vi "GE5565 Write (U64) Cluster.vi"(6 "timeout (1000 ms)":u32=1000, 8 "error in (no error)":errorcluster, 9 "buffer":dbl[](array[numeric]), 10 "offset (0)":u32, 11 "VMIC reference in":T1) -> (0 "error out":errorcluster, 3 "VMIC reference out":T1)   [LabVIEW 2015]
uses:
  <vilib>/Instr/_visa.llb/Select Event Type.ctl
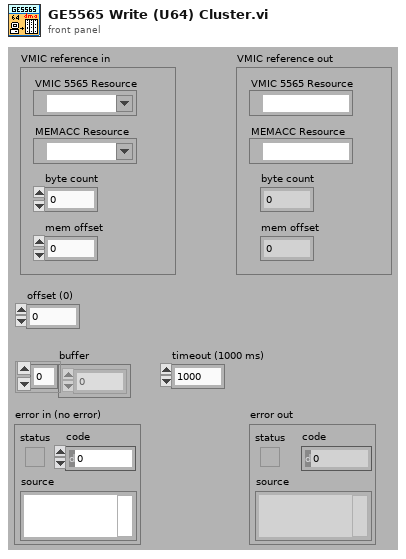
[diagram p1: front panel]
types:
  T1 = cluster{"VMIC 5565 Resource":refnum<visa-resource-name>, "MEMACC Resource":refnum<visa-resource-name>, "byte count":u32, "mem offset":u32}
  T2 = typedef "Select Event Type.ctl" = u32
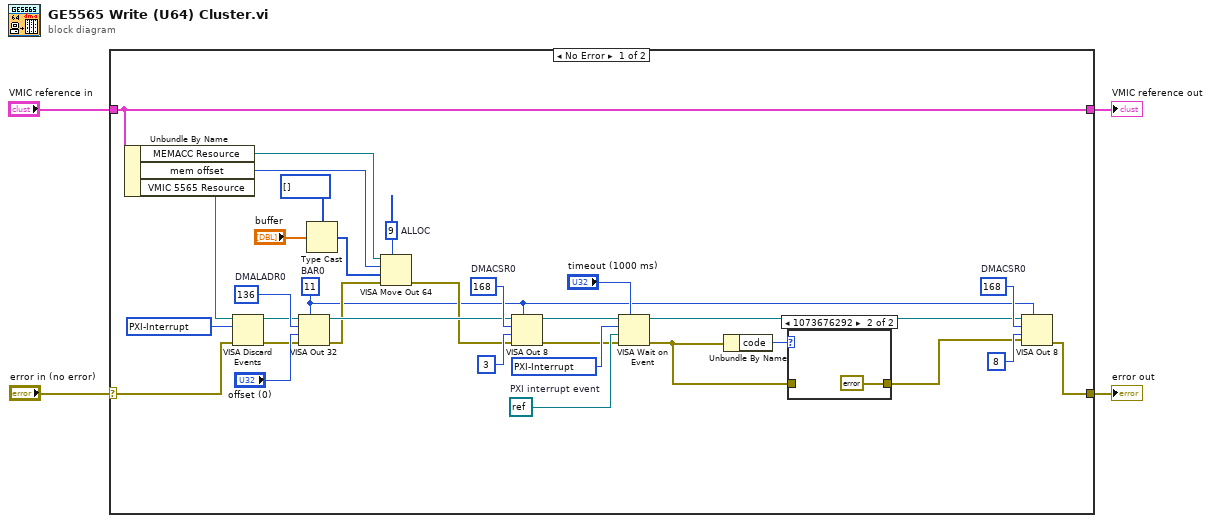
[diagram p0: block diagram]
diagram:
  n1 = case shown="No Error" "error in (no error)" {
    selector: "error in (no error)" -> [w26 w39]
    tunnel: "VMIC reference in" -> [w16 w40]
    tunnel: [w16 w40] -> w1
    tunnel: [w12 w39] -> w3
    frame No Error {
      w31 = u16 9  # ALLOC
      w13 = u16 11  # BAR0
      w28 = refnum<visa-resource-name> refnum  # PXI interrupt event
      w15 = u32 168  # DMACSR0
      w23 = T2 1073684514 items=["ServiceRequest"=1073684491, "Trigger"=3221168138, "Clear"=1073684493, "VXI-Signal"=1073684512, "VXI/VME-Interrupt"=3221168161, "VXI/VME-Sysfail"=1073684509, "VXI/VME-Sysreset"=1073684510, "GPIB-CIC"=1073684498, "GPIB-Talk"=1073684499, "GPIB-Listen"=1073684500, "PXI-Interrupt"=1073684514, "AllEnabled"=1073709055] ("Event Type")
      w29 = T2 1073684514 items=["ServiceRequest"=1073684491, "Trigger"=3221168138, "Clear"=1073684493, "VXI-Signal"=1073684512, "VXI/VME-Interrupt"=3221168161, "VXI/VME-Sysfail"=1073684509, "VXI/VME-Sysreset"=1073684510, "GPIB-CIC"=1073684498, "GPIB-Talk"=1073684499, "GPIB-Listen"=1073684500, "PXI-Interrupt"=1073684514, "AllEnabled"=1073709055] ("Event Type")
      w35 = u32 168  # DMACSR0
      w36 = u32 136  # DMALADR0
      n2 = Unbundle By Name(w16) -> ("MEMACC Resource"=w17:refnum<visa-resource-name>, "mem offset"=w18:u32, "VMIC 5565 Resource"=w20:refnum<visa-resource-name>)
      n3 = VISA Discard Events(8:w26, 10:w23, 11:w20) -> (0:w24:errorcluster, 3:w25:refnum<visa-resource-name>)  [unwired: 1 in]
      n4 = VISA Out 32(7:w13, 8:w24, 9:"offset (0)", 10:w36, 11:w25) -> (0:w19:errorcluster, 3:w33:refnum<visa-resource-name>)
      n5 = Type Cast(type=u64[] [] ("data"), x="buffer") -> (*(type *) &x=w9:u64[])
      n6 = VISA Move Out 64(7:w31, 8:w19, 9:w9, 10:w18, 11:w17) -> (0:w21:errorcluster)  [unwired: 1 out]
      n7 = VISA Out 8(7:w13, 8:w21, 9:u8 3 ("value (0)"), 10:w35, 11:w33) -> (0:w22:errorcluster, 3:w27:refnum<visa-resource-name>)
      n8 = VISA Wait on Event(7:"timeout (1000 ms)", 8:w22, 9:w28, 10:w29, 11:w27) -> (0:w8:errorcluster, 3:w7:refnum<visa-resource-name>)  [unwired: 2 out]
      n9 = Unbundle By Name(w8) -> ("code"=w5:i32)
      n10 = case shown="1073676292" w5 {
        tunnel: [w37 errorcluster {"status"=FALSE, "code"=0, "source"=""} ("error out")] -> w6
        tunnel: w8 -> [w37 _]
        frame 0, Default {
        }
        frame 1073676292 {
        }
      }
      n11 = VISA Out 8(7:w13, 8:w6, 9:u8 8 ("value (0)"), 10:w15, 11:w7) -> (0:w12:errorcluster)  [unwired: 1 out]
    }
    frame Error {
    }
  }
  "error out" <- w3
  "VMIC reference out" <- w1
